vi "Log_create_logFile_OP300-2.vi"(8 "errin":errorcluster caption="entrée d'erreur (pas d'erreur)", 10 "toute l'expression":string, 11 "Application Directory":path) -> (0 "sortie d'erreur":errorcluster, 3 "Fichier à flux d'octets en sortie":refnum<file>)   [LabVIEW 2020]
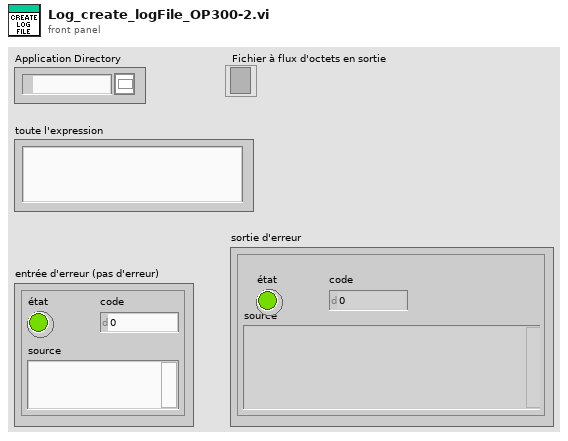
[diagram p1: front panel]
types:
  T1 = enum16{"open", "replace", "create", "open or create", "replace or create", "replace or create with confirmation"}
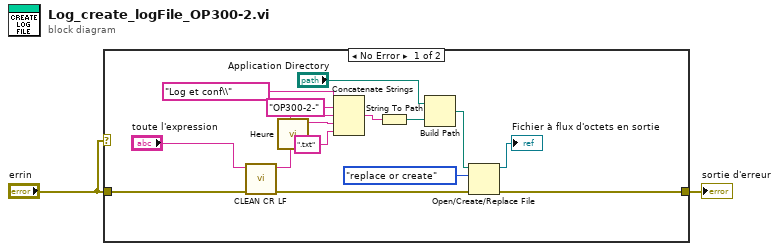
[diagram p0: block diagram]
diagram:
  n1 = case shown="No Error" "errin" {
    tunnel: [w17 w18] -> w2
    tunnel: "errin" -> [w8 w18]
    frame No Error {
      n2 = call "CLEAN CR LF.vi"("errin"=w8, "in"="toute l'expression") -> ("errout"=w7:errorcluster, "out"=w5:string)  [unwired: 8 in]
      n3 = call "Heure.vi"() -> ("chaîne concaténée"=w15:string)  [unwired: 11 in]
      n4 = Concatenate Strings("Log et conf\\", "OP300-2-" ("chaîne"), w5, w15, ".txt" ("chaîne")) -> (w13:string)
      n5 = String To Path(string=w13) -> (path=w10:path)
      n6 = Build Path(base path="Application Directory", name or relative path=w10) -> (appended path=w12:path)
      n7 = Open/Create/Replace File(file path (use dialog)=w12, error in=w7, operation (0:open)=T1."replace or create" ("opération (0 : open)")) -> (refnum out=→"Fichier à flux d'octets en sortie":refnum<file>, error out=w17:errorcluster)  [unwired: 3 in, 1 out]
    }
    frame Error {
    }
  }
  "sortie d'erreur" <- w2
